vi "Send ConfigureAppenderMsg.vi"(5 "filter":T1={"mode"=enum."Mirror", "levelMin"=enum."INFO", "levelMax"=enum."INFO", "tagPrefix"=""}, 7 "threshold":T3=enum."INFO", 8 "error in (no error)":errorcluster, 10 "id":string, 11 "Enqueuer in":refnum<class "Message Enqueuer.lvclass">) -> (0 "error out":errorcluster, 3 "Enqueuer out":refnum<class "Message Enqueuer.lvclass">)   [LabVIEW 2026, in "Lumberjack.lvlib" / "ConfigureAppenderMsg.lvclass"]
uses:
  ConfigureAppenderMsg.lvclass
  <vilib>/ActorFramework/Message Enqueuer/Message Enqueuer.lvclass
  TypeDefs/Severity.ctl
  TypeDefs/Filter.ctl
  TypeDefs/FilterMode.ctl
  ConfigureAppenderMsg.lvclass/ConfigureAppenderMsg.ctl
  <vilib>/ActorFramework/Message Enqueuer/Message Enqueuer.lvclass/Message Enqueuer.ctl
  <vilib>/ActorFramework/Message Priority Queue/Priority Enqueue.vi
  Lumberjack.lvlib
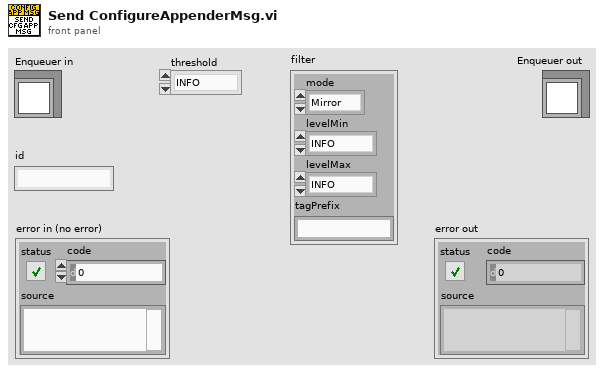
[diagram p1: front panel]
types:
  T1 = typedef "Lumberjack.lvlib/Filter.ctl" = cluster{"mode":T2, "levelMin":T3, "levelMax":T3, "tagPrefix":string}
  T2 = typedef "Lumberjack.lvlib/FilterMode.ctl" = enum16{"Mirror", "Routed"}
  T3 = typedef "Lumberjack.lvlib/Severity.ctl" = enum16{"OFF", "FATAL", "ERROR", "WARN", "INFO", "DEBUG", "TRACE", "ALL"}
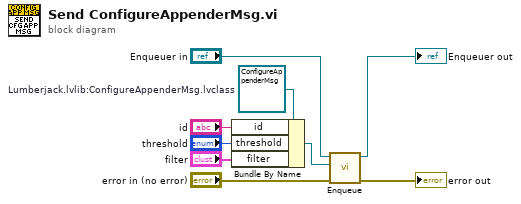
[diagram p0: block diagram]
diagram:
  w5 = refnum<class "ConfigureAppenderMsg.lvclass"> refnum  # Lumberjack.lvlib:ConfigureAppenderMsg.lvclass
  n1 = Bundle By Name(cluster=w5, "id"="id", "threshold"="threshold", "filter"="filter") -> (w3:refnum<class "ConfigureAppenderMsg.lvclass">)
  n2 = call <vilib>:"Enqueue.vi"("error in (no error)"="error in (no error)", "Message"=w3, "Message Enqueuer in"="Enqueuer in") -> ("error out"=→"error out":errorcluster, "Message Enqueuer out"=→"Enqueuer out":refnum<class "Message Enqueuer.lvclass">)  [unwired: 7 in]
